vi "Selection Handle Mouse Down.vi"(7 "Shift?":bool, 8 "error in (no error)":errorcluster, 9 "Mouse Button":u16, 10 "Mouse Coords":T1, 11 "Listbox or Tree":refnum<vi>) -> (0 "error out":errorcluster, 3 "Discard?":bool)   [LabVIEW 2020]
doc: "This VI should be called when a Mouse Down? event occurs on the <B>Listbox or Tree</B> control. Pass in the <B>Mouse Coords</B> of the event, and the <B>Shift?</B> state, and <B>Mouse Button</B> used. This VI will then change the symbols of the listbox to make it appear as if items are being selected. The output of this VI is <B>Discard?</B> which will not discard the event if he header is clicked, or if a right click operation took place.\n-------------\nBrian Hoover (hooovahh)"
uses:
  <vilib>/Utility/miscctls.llb/LVPoint32TypeDef.ctl
  Selection Global Method.ctl
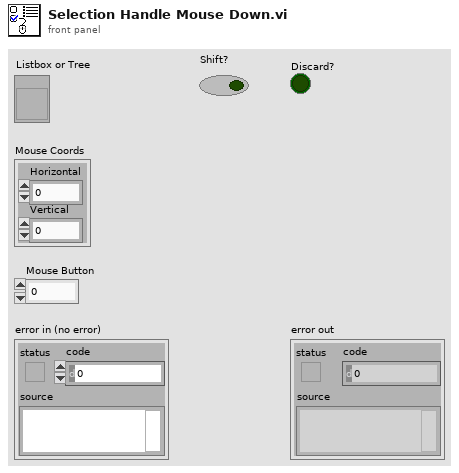
[diagram p1: front panel]
types:
  T1 = typedef "LVPoint32TypeDef.ctl" = cluster{"Horizontal":i32, "Vertical":i32}
  T2 = typedef "Selection Global Method.ctl" = enum16{"Read Selection", "Force Selection", "Mouse Down Event", "Select All", "Select None", "Invert Selection", "Read Selection and Tags"}
  T3 = typedef "LVRowAndColumnTypeDef.ctl" = cluster{"Row":i32, "Column":i32}
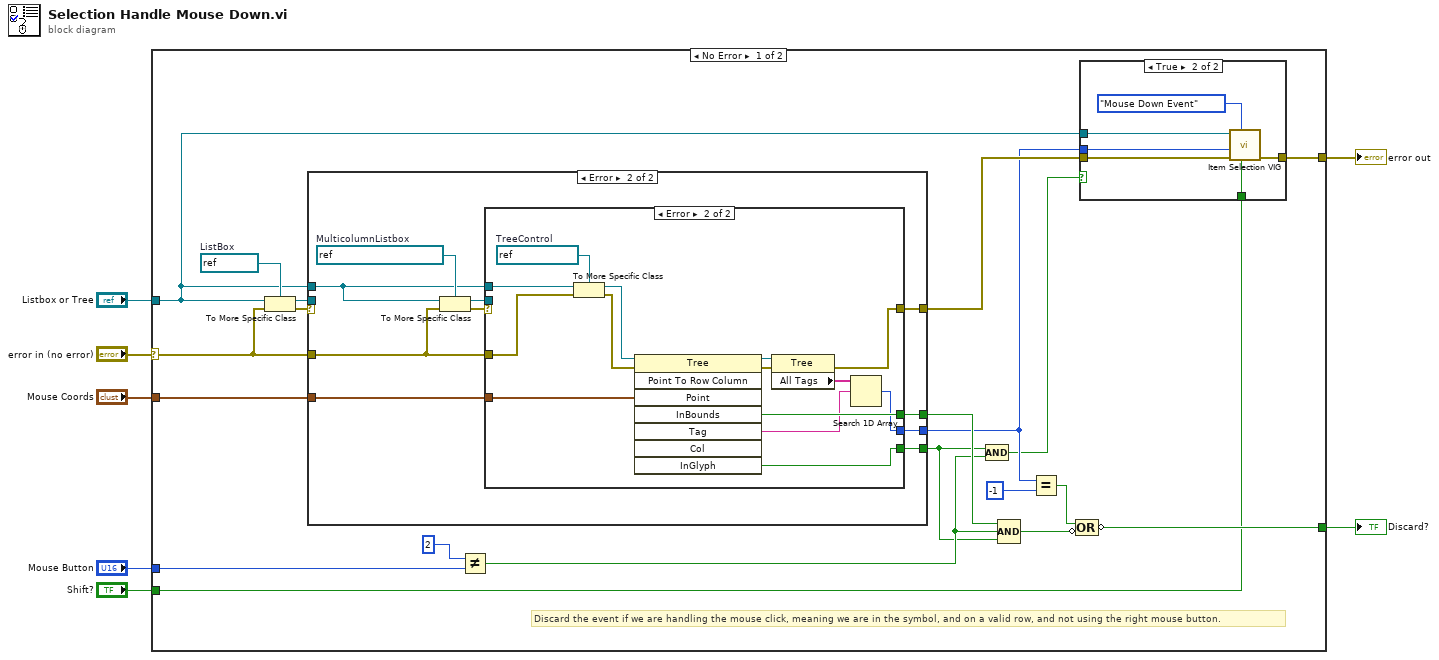
[diagram p0: block diagram]
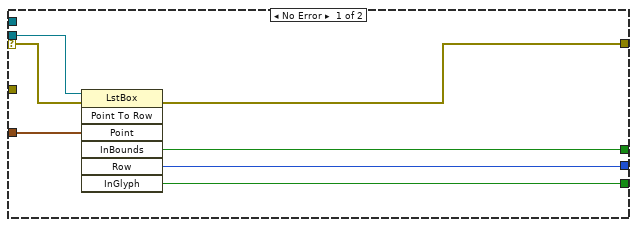
[diagram p3: hidden frame]
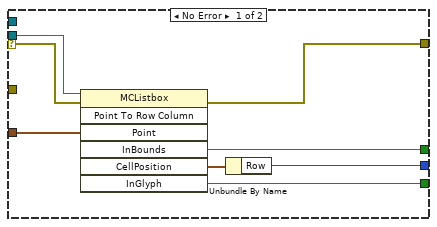
[diagram p4: hidden frame]
diagram:
  n1 = case shown="No Error" "error in (no error)" {
    selector: "error in (no error)" -> [w24 w74]
    tunnel: [w12 w74] -> w7
    tunnel: "Listbox or Tree" -> [w9 _]
    tunnel: "Mouse Coords" -> [w23 _]
    tunnel: "Mouse Button" -> [w22 _]
    tunnel: [w11 _] -> w2
    tunnel: "Shift?" -> [w10 _]
    frame No Error {
      w25 = refnum<vi> refnum  # ListBox
      # "Discard the event if we are handling the mouse click, meaning we are in the symbol, and on a valid row, and not using the right mouse button."
      n2 = To More Specific Class(target class=w25, reference=w9, error in=w24) -> (specific class reference=w27:refnum<vi>, error out=w26:errorcluster)
      n3 = case shown="Error" w26 {
        selector: w26 -> [w40 _]
        tunnel: w27 -> [w41 _]
        tunnel: w24 -> [_ w42]
        tunnel: [w39 w49] -> w15
        tunnel: w23 -> [w38 w48]
        tunnel: [w37 w46] -> w8
        tunnel: [w36 w47] -> w14
        tunnel: [w35 w45] -> w20
        tunnel: w9 -> [_ w43]
        frame No Error {
          n4 = invoke class="LstBox" method="Point To Row"(reference=w41, error in=w40, "Point"=w38) -> (error out=w39:errorcluster, "InBounds"=w35:bool, "Row"=w36:i32, "InGlyph"=w37:bool)  [unwired: 4 in, 3 out]
        }
        frame Error {
          w51 = refnum<vi> refnum  # MulticolumnListbox
          n5 = To More Specific Class(target class=w51, reference=w43, error in=w42) -> (specific class reference=w50:refnum<vi>, error out=w44:errorcluster)
          n6 = case shown="Error" w44 {
            selector: w44 -> [w52 _]
            tunnel: w50 -> [w59 _]
            tunnel: [w58 w60] -> w49
            tunnel: w48 -> [w57 w69]
            tunnel: [w55 w65] -> w47
            tunnel: [w54 w67] -> w46
            tunnel: [w53 w68] -> w45
            tunnel: w43 -> [_ w72]
            tunnel: w42 -> [_ w71]
            frame No Error {
              n7 = invoke class="MCListbox" method="Point To Row Column"(reference=w59, error in=w52, "Point"=w57) -> (error out=w58:errorcluster, "InBounds"=w53:bool, "CellPosition"=w56:T3, "InGlyph"=w54:bool)  [unwired: 4 in, 3 out]
              n8 = Unbundle By Name(w56) -> ("Row"=w55:i32)
            }
            frame Error {
              w73 = refnum<vi> refnum  # TreeControl
              n9 = To More Specific Class(target class=w73, reference=w72, error in=w71) -> (specific class reference=w64:refnum<vi>, error out=w70:errorcluster)
              n10 = invoke class="Tree" method="Point To Row Column"(reference=w64, error in=w70, "Point"=w69) -> (reference out=w63:refnum<vi>, error out=w62:errorcluster, "InBounds"=w68:bool, "Tag"=w66:string, "InGlyph"=w67:bool)  [unwired: 5 in, 3 out]
              n11 = property class="Tree"(reference=w63, error in=w62) -> (error out=w60:errorcluster, "All Tags"=w61:string[])  [unwired: 1 out]
              n12 = Search 1D Array(1D array=w61, element=w66) -> (index of element=w65:i32)  [unwired: 1 in]
            }
          }
        }
      }
      n13 = Not Equal?(x=u16 2, y=w22) -> (x != y?=w16:bool)
      n14 = Compound Arithmetic op=AND(w8, w16) -> (w13:bool)
      n15 = Compound Arithmetic op=AND(w20, w16, w8) -> (w19:bool)
      n16 = Equal?(x=w14, y=-1) -> (x = y?=w17:bool)
      n17 = Compound Arithmetic op=OR(w17, invert w19) -> (invert w11:bool)
      n18 = case shown="True" w13 {
        tunnel: w15 -> [w28 w34]
        tunnel: w9 -> [_ w33]
        tunnel: w14 -> [_ w31]
        tunnel: [w28 w30] -> w12
        tunnel: w10 -> [_ w29]
        frame False {
        }
        frame True {
          n19 = call "Item Selection VIG.vi"("Shift"=w29, "Method (Read Selection)"=Selection_Global_Method."Mouse Down Event" ("Method (Read)"), "error in (no error)"=w34, "New Selected Row"=w31, "Listbox or Tree"=w33) -> ("error out"=w30:errorcluster)  [unwired: 4 in, 2 out]
        }
      }
    }
    frame Error {
    }
  }
  "error out" <- w7
  "Discard?" <- w2
